vi "CloseDevices.vi"(8 "Stanford Err":errorcluster, 9 "Stanford ID":refnum<visa-resource-name>, 10 "Keithley Err":errorcluster, 11 "Keithley":refnum<visa-resource-name>) -> ()   [LabVIEW 2013]
uses:
  <instrlib>/Keithley 24XX/Keithley 24XX.lvlib
  <instrlib>/Stanford Research 830/Stanford Research 830.lvlib
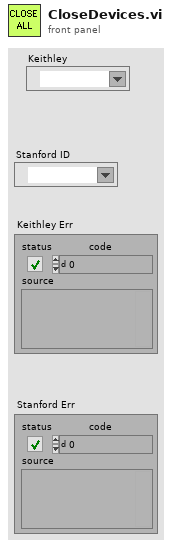
[diagram p1: front panel]
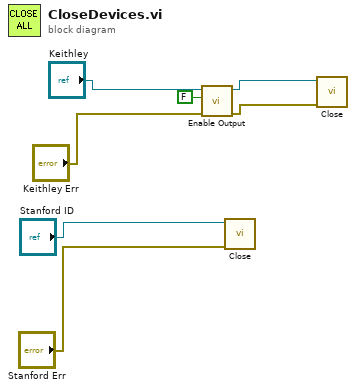
[diagram p0: block diagram]
diagram:
  n1 = call <instrlib>:"Enable Output.vi"("error in (no error)"="Keithley Err", "Enable Output (T: Enable)"=FALSE, "VISA resource name"="Keithley") -> ("error out"=w5:errorcluster, "VISA resource name out"=w6:refnum<visa-resource-name>)  [unwired: 7 in]
  n2 = call <instrlib>:"Close.vi"("error in (no error)"="Stanford Err", "VISA resource name"="Stanford ID") -> ()  [unwired: 9 in, 1 out]
  n3 = call <instrlib>:"Close.vi"("error in (no error)"=w5, "VISA resource name"=w6) -> ()  [unwired: 9 in, 1 out]
